vi "set_plot_scale_rjx.vi"(8 "set_scale":bool, 9 "rx_scale_settings":enum32{"autoscale", "fancy_scale"}(ring), 11 "plot_rjx_ref":refnum<vi>) -> ()   [LabVIEW 2025]
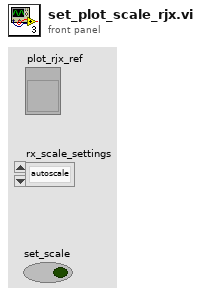
[diagram p1: front panel]
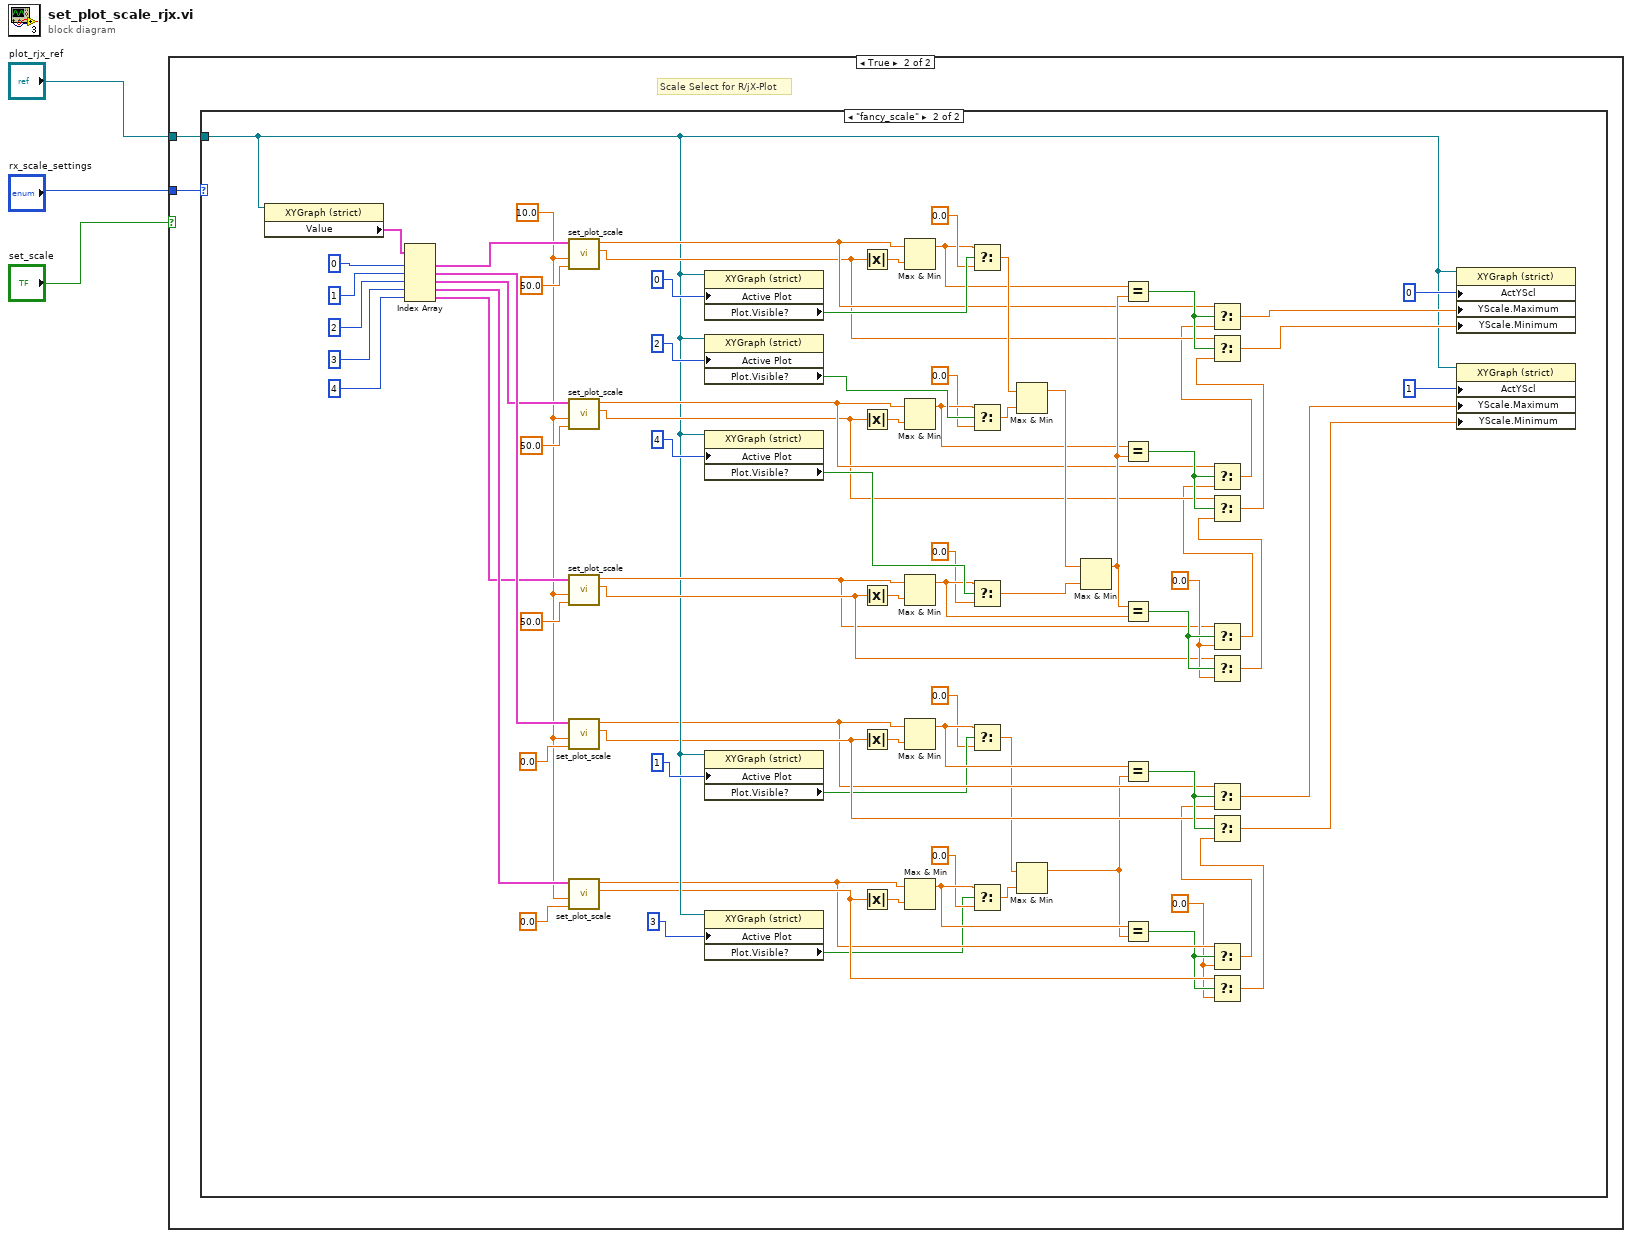
[diagram p0: block diagram]
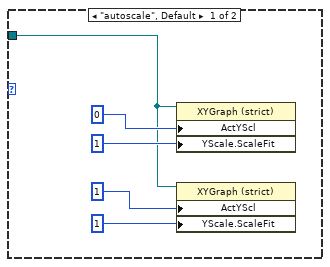
[diagram p3: hidden frame]
diagram:
  n1 = case shown="True" "set_scale" {
    tunnel: "rx_scale_settings" -> [_ w5]
    tunnel: "plot_rjx_ref" -> [_ w4]
    frame False {
    }
    frame True {
      # "Scale Select for R/jX-Plot"
      n2 = case shown="\"fancy_scale\"" w5 {
        tunnel: w4 -> [w6 w33]
        frame "autoscale", Default {
          n3 = property on="Property Node" class="XYGraph (strict)"(reference=w6, "ActYScl"=0 ("Active Y Scale"), "YScale.ScaleFit"=u8 1 ("Y Scale.Scale Fit")) -> ()  [unwired: 1 in, 2 out]
          n4 = property on="Property Node" class="XYGraph (strict)"(reference=w6, "ActYScl"=1 ("Active Y Scale"), "YScale.ScaleFit"=u8 1 ("Y Scale.Scale Fit")) -> ()  [unwired: 1 in, 2 out]
        }
        frame "fancy_scale" {
          w11 = 0.0 ("f")
          w45 = 0.0 ("t")
          w70 = 10.0 ("step")
          n5 = property class="XYGraph (strict)"(reference=w33) -> ("Value"=w88:cluster{"array type (2D Dbl)":dbl[], dbl[]}[])  [unwired: 1 in, 2 out]
          n6 = Index Array(array=w88, index #1=0 ("index"), index #2=1 ("index"), index #3=2 ("index"), index #4=3 ("index"), index #5=4 ("index")) -> (element #1=w85:cluster{"array type (2D Dbl)":dbl[], dbl[]}, element #2=w82:cluster{"array type (2D Dbl)":dbl[], dbl[]}, element #3=w77:cluster{"array type (2D Dbl)":dbl[], dbl[]}, element #4=w76:cluster{"array type (2D Dbl)":dbl[], dbl[]}, element #5=w71:cluster{"array type (2D Dbl)":dbl[], dbl[]})
          n7 = call "set_plot_scale.vi"("offset"=50.0 ("x"), "step"=w70, "plot_data"=w85) -> ("y_min"=w41:dbl, "y_max"=w42:dbl)  [unwired: 7 in]
          n8 = call "set_plot_scale.vi"("offset"=50.0 ("x"), "step"=w70, "plot_data"=w77) -> ("y_min"=w37:dbl, "y_max"=w38:dbl)  [unwired: 7 in]
          n9 = call "set_plot_scale.vi"("offset"=50.0 ("x"), "step"=w70, "plot_data"=w71) -> ("y_min"=w44:dbl, "y_max"=w43:dbl)  [unwired: 7 in]
          n10 = call "set_plot_scale.vi"("offset"=0.0 ("x"), "step"=w70, "plot_data"=w82) -> ("y_min"=w29:dbl, "y_max"=w28:dbl)  [unwired: 7 in]
          n11 = call "set_plot_scale.vi"("offset"=0.0 ("x"), "step"=w70, "plot_data"=w76) -> ("y_min"=w18:dbl, "y_max"=w17:dbl)  [unwired: 7 in]
          n12 = property on="Property Node" class="XYGraph (strict)"(reference=w33, "Active Plot"=u32 0) -> ("Plot.Visible?"=w63:bool)  [unwired: 1 in, 2 out]
          n13 = property on="Property Node" class="XYGraph (strict)"(reference=w33, "Active Plot"=u32 2) -> ("Plot.Visible?"=w60:bool)  [unwired: 1 in, 2 out]
          n14 = property on="Property Node" class="XYGraph (strict)"(reference=w33, "Active Plot"=u32 4) -> ("Plot.Visible?"=w59:bool)  [unwired: 1 in, 2 out]
          n15 = property on="Property Node" class="XYGraph (strict)"(reference=w33, "Active Plot"=u32 1) -> ("Plot.Visible?"=w27:bool)  [unwired: 1 in, 2 out]
          n16 = property on="Property Node" class="XYGraph (strict)"(reference=w33, "Active Plot"=u32 3) -> ("Plot.Visible?"=w16:bool)  [unwired: 1 in, 2 out]
          n17 = Absolute Value(x=w41) -> (abs(x)=w67:dbl)
          n18 = Absolute Value(x=w37) -> (abs(x)=w66:dbl)
          n19 = Absolute Value(x=w44) -> (abs(x)=w65:dbl)
          n20 = Absolute Value(x=w29) -> (abs(x)=w32:dbl)
          n21 = Absolute Value(x=w18) -> (abs(x)=w23:dbl)
          n22 = Max & Min(x=w42, y=w67) -> (max(x,y)=w50:dbl)  [unwired: 1 out]
          n23 = Max & Min(x=w38, y=w66) -> (max(x,y)=w49:dbl)  [unwired: 1 out]
          n24 = Max & Min(x=w43, y=w65) -> (max(x,y)=w47:dbl)  [unwired: 1 out]
          n25 = Max & Min(x=w28, y=w32) -> (max(x,y)=w30:dbl)  [unwired: 1 out]
          n26 = Max & Min(x=w17, y=w23) -> (max(x,y)=w21:dbl)  [unwired: 1 out]
          n27 = Select(t=w50, s=w63, f=0.0 ("t")) -> (s? t:f=w62:dbl)
          n28 = Select(t=w49, s=w60, f=0.0 ("t")) -> (s? t:f=w61:dbl)
          n29 = Select(t=w47, s=w59, f=0.0 ("t")) -> (s? t:f=w58:dbl)
          n30 = Select(t=w30, s=w27, f=0.0 ("t")) -> (s? t:f=w19:dbl)
          n31 = Select(t=w21, s=w16, f=0.0 ("t")) -> (s? t:f=w22:dbl)
          n32 = Max & Min(x=w62, y=w61) -> (max(x,y)=w64:dbl)  [unwired: 1 out]
          n33 = Max & Min(x=w19, y=w22) -> (max(x,y)=w15:dbl)  [unwired: 1 out]
          n34 = Max & Min(x=w64, y=w58) -> (max(x,y)=w57:dbl)  [unwired: 1 out]
          n35 = Equal?(x=w50, y=w57) -> (x = y?=w56:bool)
          n36 = Equal?(x=w49, y=w57) -> (x = y?=w55:bool)
          n37 = Equal?(x=w57, y=w47) -> (x = y?=w54:bool)
          n38 = Equal?(x=w30, y=w15) -> (x = y?=w31:bool)
          n39 = Equal?(x=w21, y=w15) -> (x = y?=w12:bool)
          n40 = Select(t=w43, s=w54, f=w45) -> (s? t:f=w36:dbl)
          n41 = Select(t=w38, s=w55, f=w36) -> (s? t:f=w40:dbl)
          n42 = Select(t=w42, s=w56, f=w40) -> (s? t:f=w52:dbl)
          n43 = Select(t=w44, s=w54, f=w45) -> (s? t:f=w35:dbl)
          n44 = Select(t=w37, s=w55, f=w35) -> (s? t:f=w39:dbl)
          n45 = Select(t=w41, s=w56, f=w39) -> (s? t:f=w53:dbl)
          n46 = Select(t=w17, s=w12, f=w11) -> (s? t:f=w14:dbl)
          n47 = Select(t=w28, s=w31, f=w14) -> (s? t:f=w25:dbl)
          n48 = Select(t=w18, s=w12, f=w11) -> (s? t:f=w13:dbl)
          n49 = Select(t=w29, s=w31, f=w13) -> (s? t:f=w24:dbl)
          n50 = property on="Property Node" class="XYGraph (strict)"(reference=w33, "ActYScl"=0 ("Active Y Scale"), "YScale.Maximum"=w52, "YScale.Minimum"=w53) -> ()  [unwired: 1 in, 2 out]
          n51 = property on="Property Node" class="XYGraph (strict)"(reference=w33, "ActYScl"=1 ("Active Y Scale"), "YScale.Maximum"=w25, "YScale.Minimum"=w24) -> ()  [unwired: 1 in, 2 out]
        }
      }
    }
  }
